vi "双向过零（乘法I8）.vi"(2 "输入":i8, 3 "复位":bool) -> (7 "双向过零":bool)   [LabVIEW 2011]
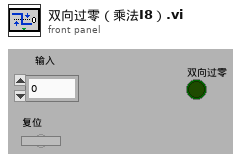
[diagram p1: front panel]
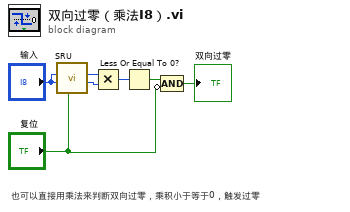
[diagram p0: block diagram]
diagram:
  # "也可以直接用乘法来判断双向过零，乘积小于等于0，触发过零"
  n1 = call-poly "SRU.vi"("复位"="复位", "初始值"="输入", "输入"="输入") -> ("本次值"=w4:i8, "上次值"=w5:i8)  [unwired: 6 in, 1 out]
  n2 = Multiply(x=w5, y=w4) -> (x*y=w3:i8)
  n3 = Less Or Equal To 0?(x=w3) -> (x <= 0?=w2:bool)
  n4 = Compound Arithmetic op=AND(w2, invert "复位") -> (→"双向过零":bool)
